vi "RPM.vi"(0 "data":dbl, 1 "factor":dbl) -> (2 "Frequency":dbl, 3 "RPM":dbl, 4 "km/h":dbl)   [LabVIEW 2014]
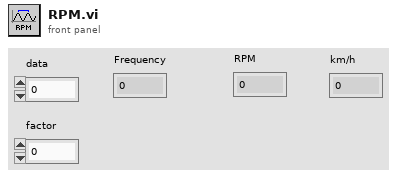
[diagram p1: front panel]
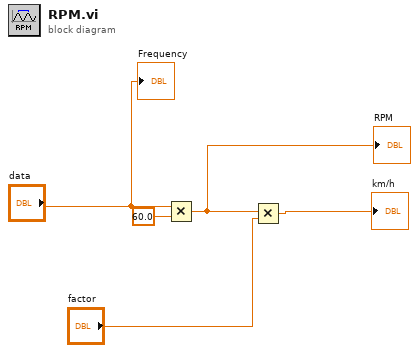
[diagram p0: block diagram]
diagram:
  n1 = Multiply(x="data", y=60.0) -> (x*y=w4:dbl)
  "RPM" <- w4
  n2 = Multiply(x=w4, y="factor") -> (x*y=→"km/h":dbl)
  "Frequency" <- "data"
